vi "Format last shot data.vi"(8 "error in (no error)":errorcluster, 11 "Shot data":T1={"Shot number"=33, "Time"=timestamp(3412282410.1945333 s since 1904-01-01), "Magnet ID"="sdqwde", "User"="sAXWCD", "Cell number"=1, "Requested field"=65.0, "Field direction"="UP", "Number of bank frames"=8, "Crowbar resistance, mOhm"=25.0, "Magnet resistance, mOhm"=35.0, "Charger voltage, kV"=9.0, "Frame voltage, kV"=10.0}) -> (0 "error out":errorcluster, 1 "Spreadsheet header string":string, 2 "Spreadsheet shot string":string, 3 "Formated shot data":string, 5 "Listbox entry":string[](array[string]))   [LabVIEW 2015]
uses:
  Shot data.ctl
  <vilib>/Utility/config.llb/NI_LVConfig.lvlib
  <vilib>/Utility/config.llb/Write Key (Boolean).vi
panel:
  in  "separator (,)":string=","
  out "Array":u32[](array[numeric])
  out "Shot data elements":string[](array[string])=["Shot number", "Time", "Magnet ID", "User", "Cell number", "Requested field", "Field direction", "Number of bank frames", "Crowbar resistance, mOhm", "Magnet resistance, mOhm", "Charger voltage, kV", "Frame voltage, kV"]
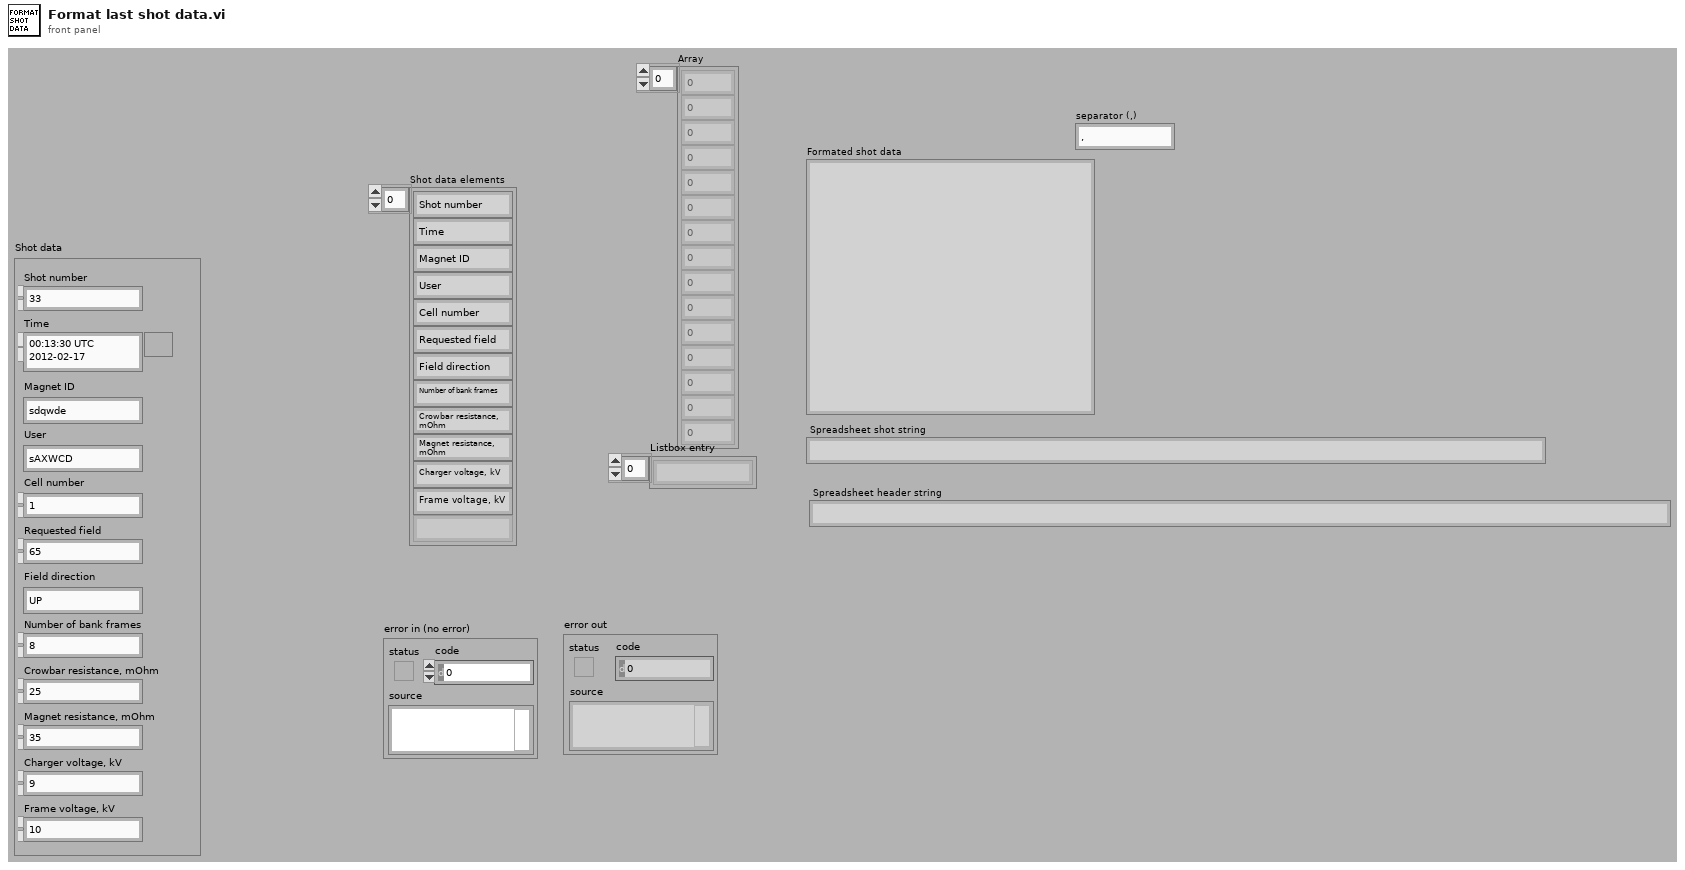
[diagram p1: front panel]
types:
  T1 = typedef "Shot data.ctl" = cluster{"Shot number":i32, "Time":timestamp, "Magnet ID":string, "User":string, "Cell number":i32, "Requested field":dbl, "Field direction":string, "Number of bank frames":i32, "Crowbar resistance, mOhm":dbl, "Magnet resistance, mOhm":dbl, "Charger voltage, kV":dbl, "Frame voltage, kV":dbl}
  T2 = cluster{"[0]":string, "[1]":string, "[2]":string, "[3]":string, "[4]":string, "[5]":string, "[6]":string, "[7]":string, "[8]":string, "[9]":string, "[10]":string, "[11]":string}
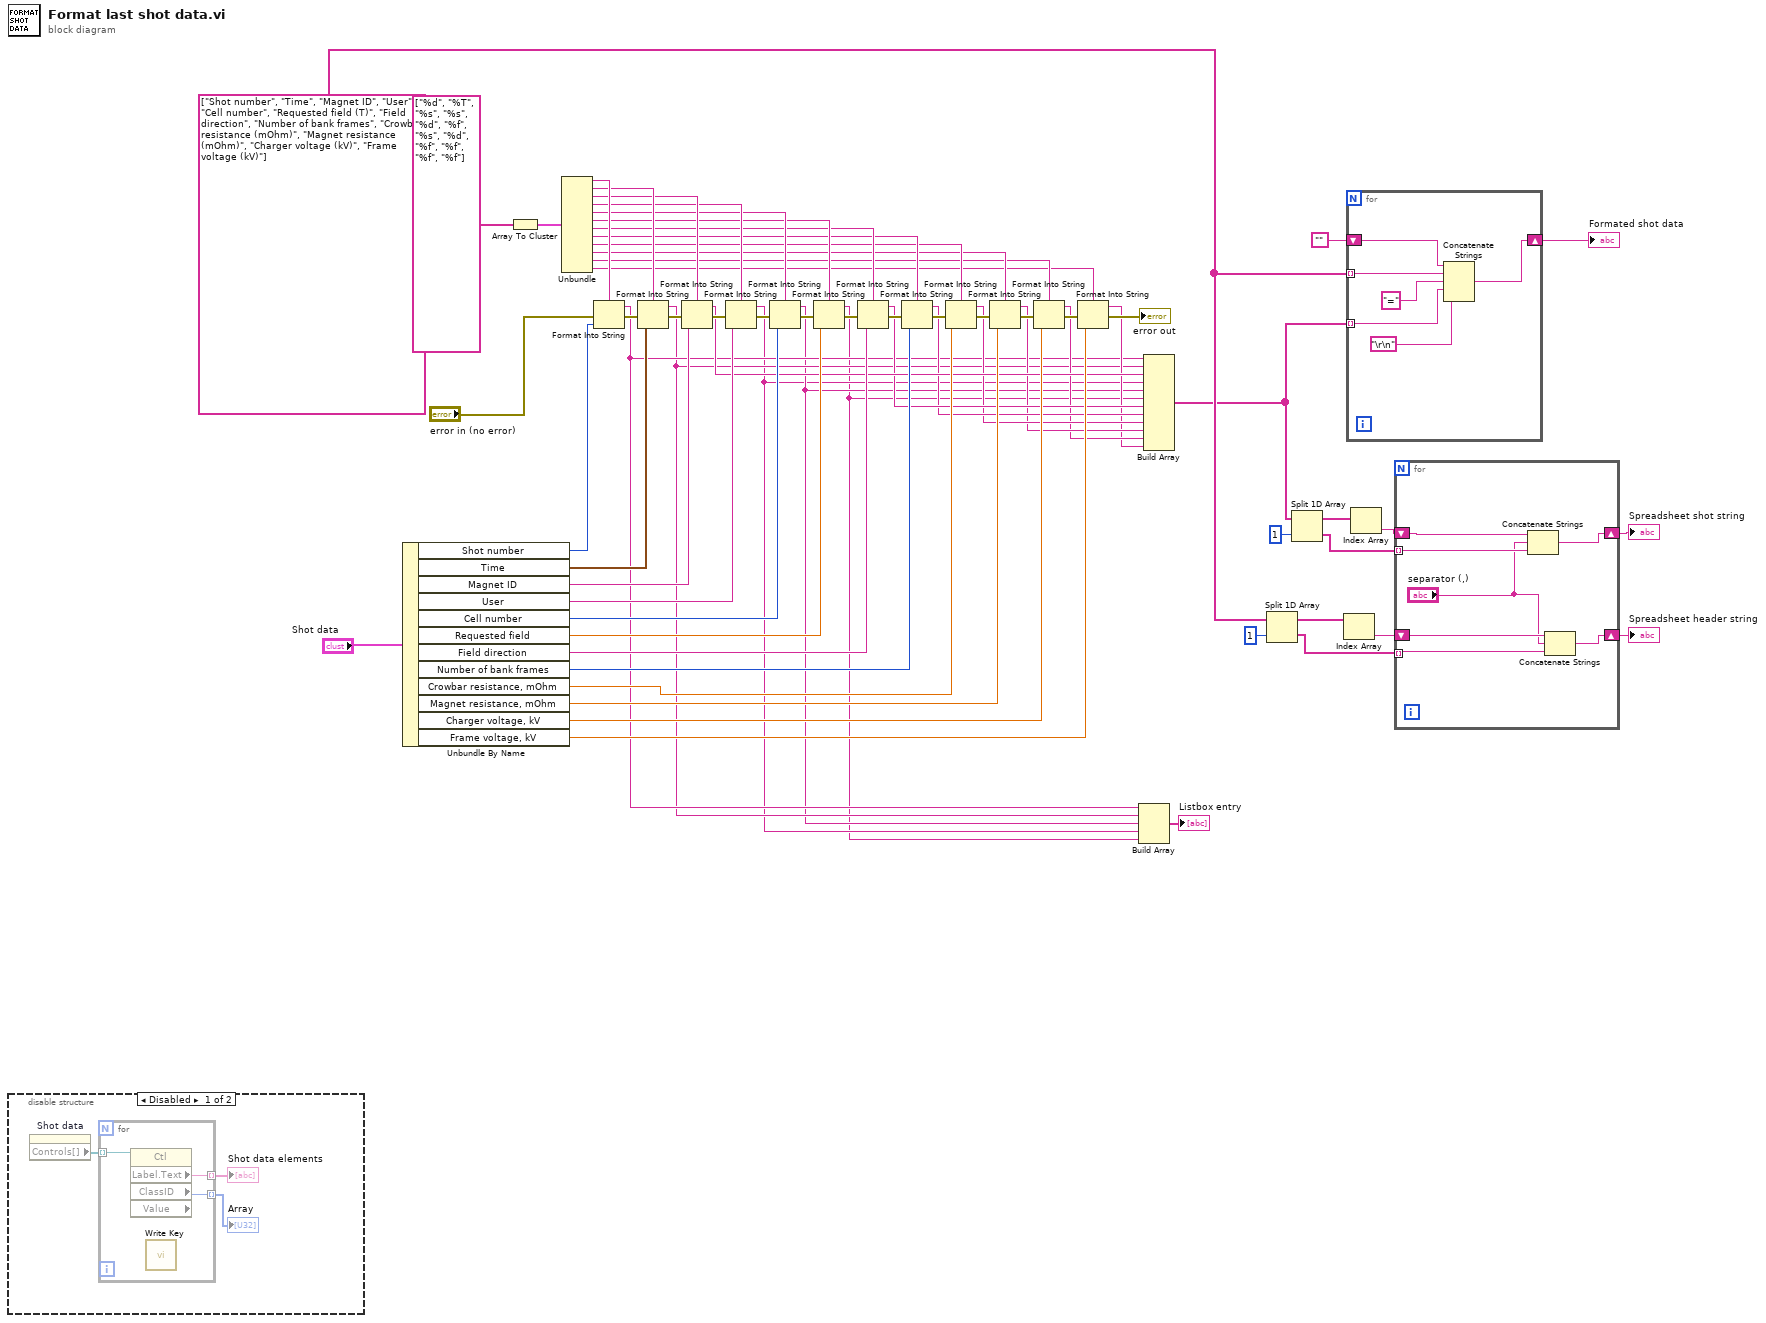
[diagram p0: block diagram]
diagram:
  w8 = string[] ["Shot number", "Time", "Magnet ID", "User", "Cell number", "Requested field (T)", "Field direction", "Number of bank frames", "Crowbar resistance (mOhm)", "Magnet resistance (mOhm)", "Charger voltage (kV)", "Frame voltage (kV)"] ("Shot data elements")
  n1 = disable-structure shown="Disabled" {
    frame Disabled {
      n2 = property on="Shot data" class="Clust (strict)"() -> ("Controls[]"=w70:refnum<vi>[])  [unwired: 2 in, 2 out]
      n3 = for {
        tunnel: w70 -> [w73] mode=indexing
        tunnel: [w72] -> w69 mode=indexing
        tunnel: [w71] -> w68 mode=indexing
        n4 = property class="Ctl" props=["Label", "Text", "ClassID", "Value"](reference=w73) -> ("Label.Text"=w72:string, "ClassID"=w71:u32)  [unwired: 1 in, 3 out]
        n5 = call-poly <vilib>:"Write Key.vi"() -> ()  [unwired: 9 in, 3 out]
      }
      "Shot data elements" <- w69
      "Array" <- w68
    }
    frame Enabled {
    }
  }
  n6 = Unbundle By Name("Shot data") -> ("Shot number"=w53:i32, "Time"=w52:timestamp, "Magnet ID"=w51:string, "User"=w50:string, "Cell number"=w49:i32, "Requested field"=w48:dbl, "Field direction"=w47:string, "Number of bank frames"=w46:i32, "Crowbar resistance, mOhm"=w45:dbl, "Magnet resistance, mOhm"=w44:dbl, "Charger voltage, kV"=w43:dbl, "Frame voltage, kV"=w42:dbl)
  n7 = Array To Cluster(array=string[] ["%d", "%T", "%s", "%s", "%d", "%f", "%s", "%d", "%f", "%f", "%f", "%f"]) -> (cluster=w41:T2)
  n8 = Unbundle(w41) -> ("[0]"=w39:string, "[1]"=w38:string, "[2]"=w37:string, "[3]"=w36:string, "[4]"=w35:string, "[5]"=w34:string, "[6]"=w33:string, "[7]"=w32:string, "[8]"=w31:string, "[9]"=w30:string, "[10]"=w29:string, "[11]"=w28:string)
  n9 = Format Into String(format string=w39, error in="error in (no error)", w53) -> (resulting string=w6:string, error out=w66:errorcluster)  [unwired: 1 in]
  n10 = Format Into String(format string=w38, error in=w66, w52) -> (resulting string=w5:string, error out=w65:errorcluster)  [unwired: 1 in]
  n11 = Format Into String(format string=w37, error in=w65, w51) -> (resulting string=w27:string, error out=w64:errorcluster)  [unwired: 1 in]
  n12 = Format Into String(format string=w36, error in=w64, w50) -> (resulting string=w3:string, error out=w63:errorcluster)  [unwired: 1 in]
  n13 = Format Into String(format string=w35, error in=w63, w49) -> (resulting string=w4:string, error out=w62:errorcluster)  [unwired: 1 in]
  n14 = Format Into String(format string=w34, error in=w62, w48) -> (resulting string=w2:string, error out=w61:errorcluster)  [unwired: 1 in]
  n15 = Format Into String(format string=w33, error in=w61, w47) -> (resulting string=w26:string, error out=w60:errorcluster)  [unwired: 1 in]
  n16 = Format Into String(format string=w32, error in=w60, w46) -> (resulting string=w25:string, error out=w59:errorcluster)  [unwired: 1 in]
  n17 = Format Into String(format string=w31, error in=w59, w45) -> (resulting string=w24:string, error out=w57:errorcluster)  [unwired: 1 in]
  n18 = Format Into String(format string=w30, error in=w57, w44) -> (resulting string=w23:string, error out=w58:errorcluster)  [unwired: 1 in]
  n19 = Format Into String(format string=w29, error in=w58, w43) -> (resulting string=w22:string, error out=w56:errorcluster)  [unwired: 1 in]
  n20 = Format Into String(format string=w28, error in=w56, w42) -> (resulting string=w21:string, error out=→"error out":errorcluster)  [unwired: 1 in]
  n21 = Build Array(w6, w5, w4, w3, w2) -> (→"Listbox entry":string[])
  n22 = Build Array(w6, w5, w27, w3, w4, w2, w26, w25, w24, w23, w22, w21) -> (w7:string[])
  n23 = Split 1D Array(array=w8, index=1) -> (first subarray=w16:string[], second subarray=w11:string[])
  n24 = Split 1D Array(array=w7, index=1) -> (first subarray=w13:string[], second subarray=w10:string[])
  n25 = Index Array(array=w16) -> (element=w15:string)  [unwired: 1 in]
  n26 = for {
    tunnel: w8 -> [w79] mode=indexing
    tunnel: w7 -> [w77] mode=indexing
    shift-right: [w74] -> w20
    shift-left: "" -> [w75]
    n27 = Concatenate Strings(w75, w79, "=", w77, "\r\n") -> (w74:string)
  }
  "Formated shot data" <- w20
  n28 = Index Array(array=w13) -> (element=w12:string)  [unwired: 1 in]
  n29 = for {
    shift-right: [w84] -> w18
    shift-left: w12 -> [w86]
    tunnel: w10 -> [w85] mode=indexing
    shift-right: [w80] -> w14
    shift-left: w15 -> [w83]
    tunnel: w11 -> [w81] mode=indexing
    n30 = Concatenate Strings(w86, "separator (,)", w85) -> (w84:string)
    n31 = Concatenate Strings(w83, "separator (,)", w81) -> (w80:string)
  }
  "Spreadsheet shot string" <- w18
  "Spreadsheet header string" <- w14
